vi "Autonomous Independent.vi"() -> ()   [LabVIEW 2014]
doc: "This VI is called when autonomous begins, and will automatically be terminated when autonomous ends. You can carry out timed or sensor driven robot movement independently without needing to return to the caller."
uses:
  <vilib>/Rock Robotics/WPI/CAN/TalonSRX/WPI_CANTalonSRX_APIControlMode.ctl
  <vilib>/Rock Robotics/WPI/Joystick/WPI_JoystickGetSetRefNum.vi
  Robot Global Data.vi
  <vilib>/Rock Robotics/WPI/RobotDrive/WPI_RobotDriveArcadeDrive_Standard(NoSaturation).vi
panel:
  out "Applied Throttle 2":dbl[](graph)
  out "Encoder Graph 2":dbl[](graph)
  in  "Numeric 2":dbl=1000.0 format="%#_13g"
  in  "Numeric":dbl=1000.0 format="%#_13g"
  out "Encoder Graph":dbl[](graph)
  out "Applied Throttle":dbl[](graph)
  out "Current Movement, for debugging":T1 {"Y Joystick Value" scale=1.0..-1.0; "X Joystick Value" scale=-1.0..1.0}
  in  "Array of robot movements":T2(array[cluster]) {"Y Joystick Value" scale=1.0..-1.0; "X Joystick Value" scale=-1.0..1.0}
  # "Be sure to right-click and choose Data Operations>>Make Current Value default if you want to save the array values with the VI"
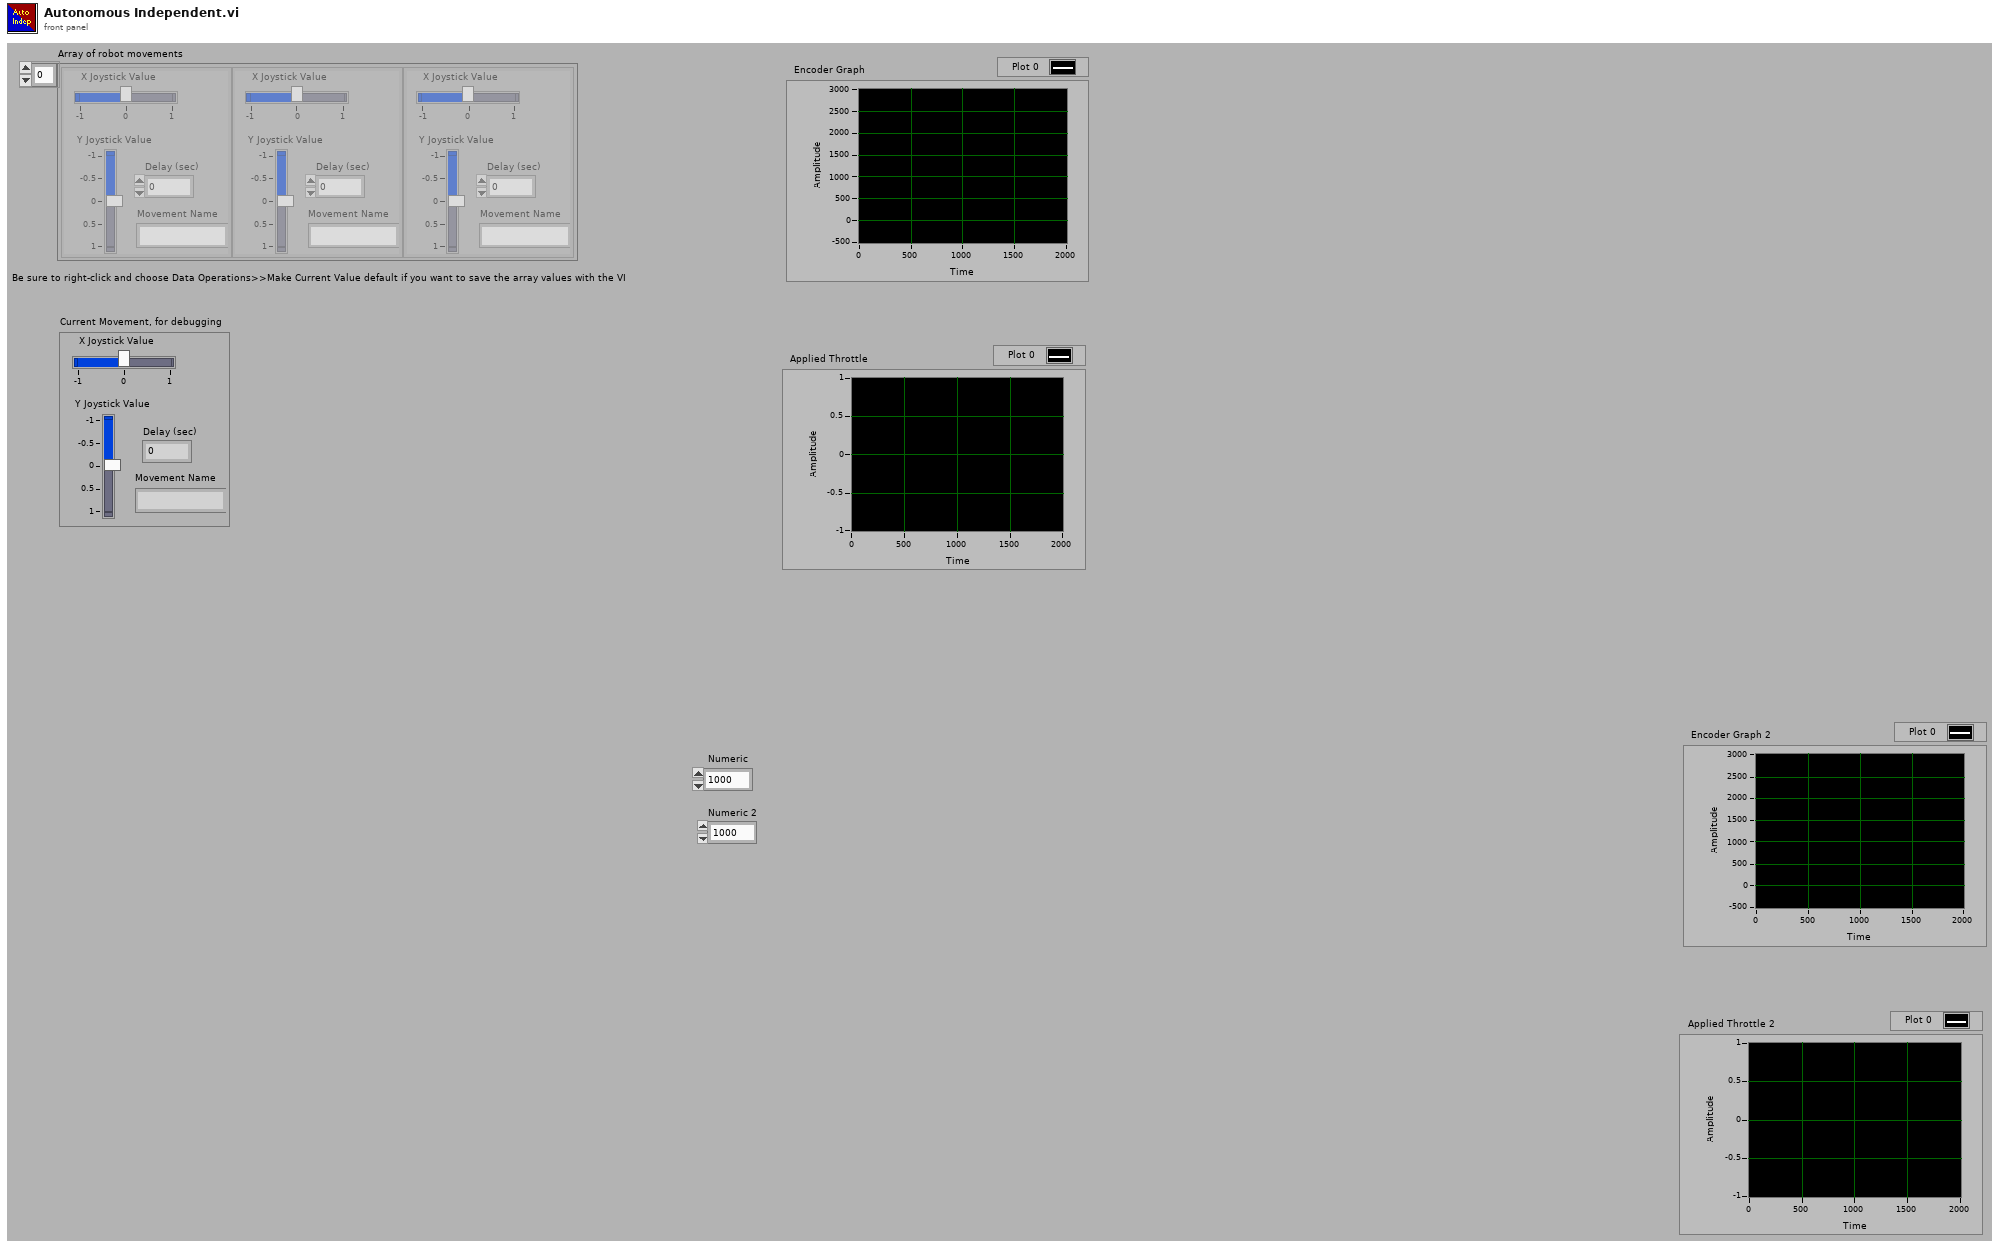
[diagram p1: front panel]
types:
  T1 = cluster{"X Joystick Value":dbl, "Y Joystick Value":dbl, "Delay (sec)":dbl, "Movement Name":string}
  T2 = cluster{"X Joystick Value":dbl, "Y Joystick Value":dbl, "Delay (sec)":dbl, "Movement Name":string}[]
  T3 = typedef "WPI_CANTalonSRX_APIControlMode.ctl" = enum8{"Percent VBus", "Speed", "Position", "Slave", "Unchanged / Invalid"}
  T4 = cluster{"proportional gain (Kc)":dbl, "integral time (Ti, min)":dbl, "derivative time (Td, min)":dbl}
  T5 = typedef "WPI_MotorControlDeviceRef.ctl" = cluster{"DeviceStatus":errorcluster, "Type":T6, "PWM":cluster{"Controller":T7, "PWM Channel":T8, "DeadBand":T9}, "CAN":cluster{"Device Number":u8, "Control Mode":T10, "Semaphore":T11, "Max Vout":dbl, "TalonSRX Control Mode":T3}, "Invert":bool, "TransformRef":T12, "InvTransformRef":T12}
  T6 = typedef "WPI_MotorControlType.ctl" = enum16{"PWM", "CAN", "CANTalonSRX"}
  T7 = typedef "FPGA_TypedefDigitalModule.ctl" = enum16{"Controller 1"}
  T8 = typedef "FPGA_DIOPWMChannel.ctl" = enum8{"PWM 0", "PWM 1", "PWM 2", "PWM 3", "PWM 4", "PWM 5", "PWM 6", "PWM 7", "PWM 8", "PWM 9", "PWM MXP 0", "PWM MXP 1", "PWM MXP 2", "PWM MXP 3", "PWM MXP 4", "PWM MXP 5", "PWM MXP 6", "PWM MXP 7", "PWM MXP 8", "PWM MXP 9", "Invalid"}
  T9 = typedef "WPI_PWMDeadband.ctl" = cluster{"Name":string, "maxPositivePwm":i32, "minPositivePwm":i32, "centerPwm":i32, "maxNegativePwm":i32, "minNegativePwm":i32, "angularRange":u16}
  T10 = typedef "WPI_CANJaguar_ControlMode.ctl" = enum8{"Percent VBus", "Current", "Speed", "Position", "Voltage"}
  T11 = typedef "Semaphore RefNum" = refnum<k1>
  T12 = typedef "WPI_PWMTransform_ConPane.ctl" = refnum<vi>
  T13 = typedef "WPI_CANTalonSRX_GlobalStatus.ctl" = cluster{"Applied Throttle":dbl, "Module Enabled":bool, "CAN Error":errorcluster, "Closed Loop Error":dbl, "Forward Limit Switch Closed":bool, "Reverse Limit Switch Closed":bool, "Sensor Position":dbl, "Sensor Velocity":dbl, "Current":dbl, "Sticky Fault - Over Temp":bool, "Sticky Fault - Under Voltage":bool, "Sticky Fault - Forward Limit":bool, "Sticky Fault - Reverse Limit":bool, "Sticky Fault - Forward Soft Limit":bool, "Sticky Fault - Reverse Soft Limit":bool, "Brake is Enabled":bool, "Encoder Position":dbl, "Encoder Velocity":dbl, "Encoder Index Count":dbl, "Encoder A Pin State":bool, "Encoder B Pin State":bool, "Encoder Index Pin State":bool, "Analog In":dbl, "Analog In Velocity":dbl, "Temperature (C)":dbl, "Battery Voltage":dbl}
  T14 = typedef "WPI_RobotDriveDevRef.ctl" = cluster{"DevStatus":errorcluster, "Motors[]":T5[], "Square Inputs":bool, "Max Output":dbl}
  T15 = typedef "WPI_EncoderDevRef.ctl" = cluster{"DevStatus":errorcluster, "EncoderIndex":T16, "CounterIndex":T17, "DistancePerCount":dbl, "Decoding Type":T18}
  T16 = typedef "FPGA_EncoderIdx.ctl" = enum8{"Enc 0", "Enc 1", "Enc 2", "Enc 3", "Enc 4", "Enc 5", "Enc 6", "Enc 7", "Invalid"}
  T17 = typedef "FPGA_CounterCtrSystemIndex.ctl" = enum8{"Ctr 0", "Ctr 1", "Ctr 2", "Ctr 3", "Ctr 4", "Ctr 5", "Ctr 6", "Ctr 7", "Invalid"}
  T18 = typedef "WPI_EncoderType.ctl" = enum16{"1x", "2x", "4x"}
  T19 = typedef "WPI_JoystickDevRef.ctl" = cluster{"Device":T20}
  T20 = typedef "WPI_JoystickDeviceEnum.ctl" = enum16{"USB 0", "USB 1", "USB 2", "USB 3", "USB 4", "USB 5"}
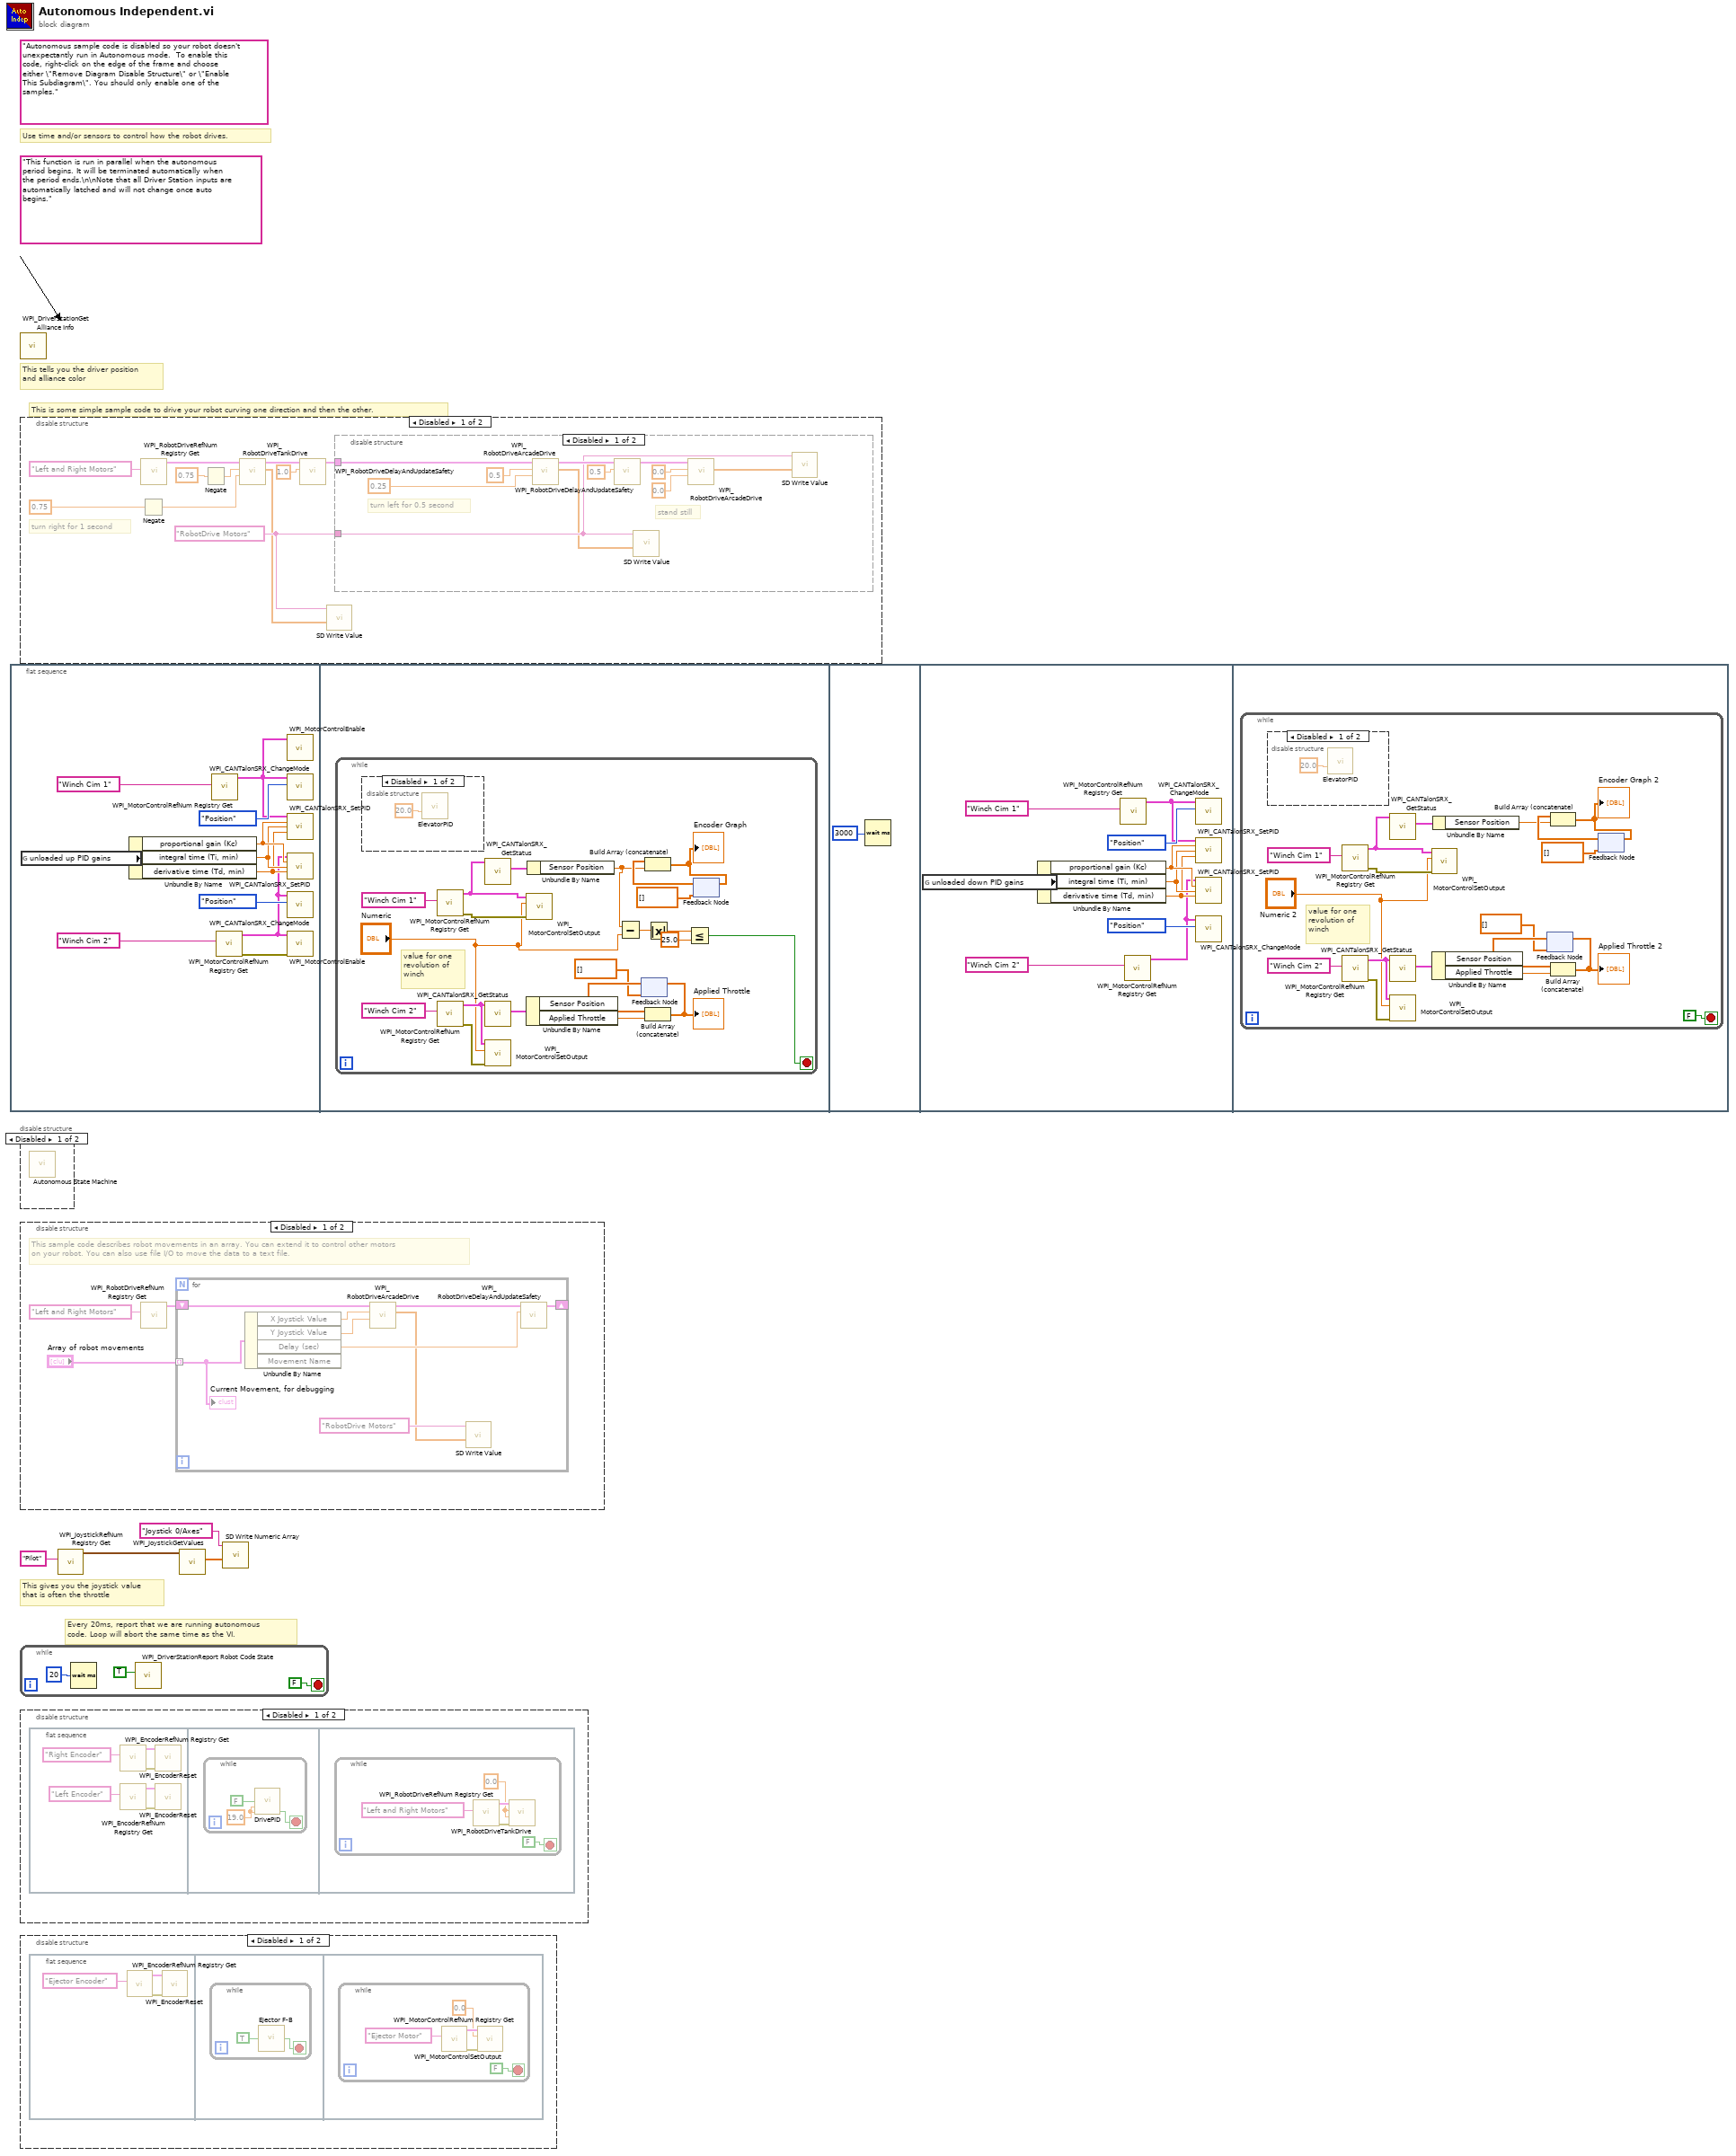
[diagram p0: block diagram]
diagram:
  (unwired) "Autonomous sample code is disabled so your robot doesn't unexpectantly run in Autonomous mode.  To enable this code, right-click on the edge of the frame and choose either \"Remove Diagram Disable Structure\" or \"Enable This Subdiagram\". You should only enable one of the samples."
  (unwired) "This function is run in parallel when the autonomous period begins. It will be terminated automatically when the period ends.\n\nNote that all Driver Station inputs are automatically latched and will not change once auto begins."
  # "This is some simple sample code to drive your robot curving one direction and then the other."
  # "Every 20ms, report that we are running autonomous\ncode. Loop will abort the same time as the VI."
  # "This gives you the joystick value\nthat is often the throttle"
  # "Use time and/or sensors to control how the robot drives."
  # "This tells you the driver position\nand alliance color"
  n1 = flat-sequence {
    frame #0 {
      n2 = global read "Robot Global Data.vi" "unloaded up PID gains"() -> (w10:T4)
      n3 = Unbundle By Name(w10) -> ("proportional gain (Kc)"=w9:dbl, "integral time (Ti, min)"=w8:dbl, "derivative time (Td, min)"=w7:dbl)
      n4 = call <vilib>:"WPI_MotorControlRefNum Registry Get.vi"("refnum name"="Winch Cim 1") -> ("MotorControlDevRef"=w5:T5)  [unwired: 9 in, 1 out]
      n5 = call <vilib>:"WPI_MotorControlRefNum Registry Get.vi"("refnum name"="Winch Cim 2") -> ("error out"=w14:errorcluster, "MotorControlDevRef"=w6:T5)  [unwired: 9 in]
      n6 = call <vilib>:"WPI_MotorControlEnable.vi"("CAN Jaguar Ref"=w5) -> ()  [unwired: 9 in, 2 out]
      n7 = call <vilib>:"WPI_CANTalonSRX_ChangeMode.vi"("Control Mode"=WPI_CANTalonSRX_APIControlMode."Position", "CAN Talon SRX Ref"=w5) -> ()  [unwired: 8 in, 2 out]
      n8 = call <vilib>:"WPI_CANTalonSRX_SetPID.vi"("CAN Talon SRX Ref"=w5, "P"=w9, "I"=w8, "D"=w7) -> ()  [unwired: 10 in, 2 out]
      n9 = call <vilib>:"WPI_CANTalonSRX_SetPID.vi"("CAN Talon SRX Ref"=w6, "P"=w9, "I"=w8, "D"=w7) -> ()  [unwired: 10 in, 2 out]
      n10 = call <vilib>:"WPI_CANTalonSRX_ChangeMode.vi"("Control Mode"=WPI_CANTalonSRX_APIControlMode."Position", "CAN Talon SRX Ref"=w6) -> ()  [unwired: 8 in, 2 out]
      n11 = call <vilib>:"WPI_MotorControlEnable.vi"("error in (no error)"=w14, "CAN Jaguar Ref"=w6) -> ()  [unwired: 8 in, 2 out]
    }
    frame #1 {
      n12 = while {
        stop <- w16 stop-if-true
        # "value for one \nrevolution of \nwinch"
        n13 = disable-structure shown="Disabled" {
          frame Disabled {
            n14 = call "ElevatorPID.vi"("Elevator Setpoint"=20.0 ("SetpointLeft")) -> ()  [unwired: 14 in, 1 out]
          }
          frame Enabled {
          }
        }
        n15 = call <vilib>:"WPI_MotorControlRefNum Registry Get.vi"("refnum name"="Winch Cim 1") -> ("error out"=w34:errorcluster, "MotorControlDevRef"=w32:T5)  [unwired: 9 in]
        n16 = call <vilib>:"WPI_MotorControlRefNum Registry Get.vi"("refnum name"="Winch Cim 2") -> ("error out"=w33:errorcluster, "MotorControlDevRef"=w31:T5)  [unwired: 9 in]
        n17 = call <vilib>:"WPI_CANTalonSRX_GetStatus.vi"("CAN Talon SRX Ref"=w32) -> ("Talon SRX Status"=w30:T13)  [unwired: 8 in, 2 out]
        n18 = call <vilib>:"WPI_CANTalonSRX_GetStatus.vi"("CAN Talon SRX Ref"=w31) -> ("Talon SRX Status"=w22:T13)  [unwired: 8 in, 2 out]
        n19 = call <vilib>:"WPI_MotorControlSetOutput.vi"("error in (no error)"=w33, "Output"="Numeric", "MotorControlDevRef"=w31) -> ()  [unwired: 6 in, 3 out]
        n20 = call <vilib>:"WPI_MotorControlSetOutput.vi"("error in (no error)"=w34, "Output"="Numeric", "MotorControlDevRef"=w32) -> ()  [unwired: 6 in, 3 out]
        n21 = Unbundle By Name(w22) -> ("Applied Throttle"=w24:dbl)  [unwired: 1 out]
        n22 = Unbundle By Name(w30) -> ("Sensor Position"=w21:dbl)
        n23 = Subtract(x=w21, y="Numeric") -> (x-y=w19:dbl)
        n24 = feedback #1(dbl[] []) -> (w29:dbl[])
        n25 = Build Array (concatenate)(w29, w24) -> (w23:dbl[])
        "Applied Throttle" <- w23
        n26 = feedback-in #1(w23) -> ()
        n27 = Absolute Value(x=w19) -> (abs(x)=w18:dbl)
        n28 = Less Or Equal?(x=w18, y=25.0) -> (x <= y?=w16:bool)
        n29 = feedback #2(dbl[] []) -> (w26:dbl[])
        n30 = Build Array (concatenate)(w26, w21) -> (w27:dbl[])
        "Encoder Graph" <- w27
        n31 = feedback-in #2(w27) -> ()
      }
    }
    frame #2 {
      n32 = Wait (ms)(milliseconds to wait=u32 3000) -> ()  [unwired: 1 out]
    }
    frame #3 {
      n33 = global read "Robot Global Data.vi" "unloaded down PID gains"() -> (w44:T4)
      n34 = Unbundle By Name(w44) -> ("proportional gain (Kc)"=w43:dbl, "integral time (Ti, min)"=w42:dbl, "derivative time (Td, min)"=w41:dbl)
      n35 = call <vilib>:"WPI_MotorControlRefNum Registry Get.vi"("refnum name"="Winch Cim 1") -> ("MotorControlDevRef"=w39:T5)  [unwired: 9 in, 1 out]
      n36 = call <vilib>:"WPI_MotorControlRefNum Registry Get.vi"("refnum name"="Winch Cim 2") -> ("MotorControlDevRef"=w40:T5)  [unwired: 9 in, 1 out]
      n37 = call <vilib>:"WPI_CANTalonSRX_ChangeMode.vi"("Control Mode"=WPI_CANTalonSRX_APIControlMode."Position", "CAN Talon SRX Ref"=w39) -> ()  [unwired: 8 in, 2 out]
      n38 = call <vilib>:"WPI_CANTalonSRX_SetPID.vi"("CAN Talon SRX Ref"=w39, "P"=w43, "I"=w42, "D"=w41) -> ()  [unwired: 10 in, 2 out]
      n39 = call <vilib>:"WPI_CANTalonSRX_SetPID.vi"("CAN Talon SRX Ref"=w40, "P"=w43, "I"=w42, "D"=w41) -> ()  [unwired: 10 in, 2 out]
      n40 = call <vilib>:"WPI_CANTalonSRX_ChangeMode.vi"("Control Mode"=WPI_CANTalonSRX_APIControlMode."Position", "CAN Talon SRX Ref"=w40) -> ()  [unwired: 8 in, 2 out]
    }
    frame #4 {
      n41 = while {
        stop <- FALSE stop-if-true
        # "value for one \nrevolution of \nwinch"
        n42 = disable-structure shown="Disabled" {
          frame Disabled {
            n43 = call "ElevatorPID.vi"("Elevator Setpoint"=20.0 ("SetpointLeft")) -> ()  [unwired: 14 in, 1 out]
          }
          frame Enabled {
          }
        }
        n44 = call <vilib>:"WPI_MotorControlRefNum Registry Get.vi"("refnum name"="Winch Cim 1") -> ("error out"=w63:errorcluster, "MotorControlDevRef"=w61:T5)  [unwired: 9 in]
        n45 = call <vilib>:"WPI_MotorControlRefNum Registry Get.vi"("refnum name"="Winch Cim 2") -> ("error out"=w62:errorcluster, "MotorControlDevRef"=w60:T5)  [unwired: 9 in]
        n46 = call <vilib>:"WPI_CANTalonSRX_GetStatus.vi"("CAN Talon SRX Ref"=w61) -> ("Talon SRX Status"=w59:T13)  [unwired: 8 in, 2 out]
        n47 = call <vilib>:"WPI_CANTalonSRX_GetStatus.vi"("CAN Talon SRX Ref"=w60) -> ("Talon SRX Status"=w51:T13)  [unwired: 8 in, 2 out]
        n48 = call <vilib>:"WPI_MotorControlSetOutput.vi"("error in (no error)"=w62, "Output"="Numeric 2", "MotorControlDevRef"=w60) -> ()  [unwired: 6 in, 3 out]
        n49 = call <vilib>:"WPI_MotorControlSetOutput.vi"("error in (no error)"=w63, "Output"="Numeric 2", "MotorControlDevRef"=w61) -> ()  [unwired: 6 in, 3 out]
        n50 = Unbundle By Name(w51) -> ("Applied Throttle"=w53:dbl)  [unwired: 1 out]
        n51 = Unbundle By Name(w59) -> ("Sensor Position"=w50:dbl)
        n52 = feedback #3(dbl[] []) -> (w58:dbl[])
        n53 = Build Array (concatenate)(w58, w53) -> (w52:dbl[])
        "Applied Throttle 2" <- w52
        n54 = feedback-in #3(w52) -> ()
        n55 = feedback #4(dbl[] []) -> (w55:dbl[])
        n56 = Build Array (concatenate)(w55, w50) -> (w56:dbl[])
        "Encoder Graph 2" <- w56
        n57 = feedback-in #4(w56) -> ()
      }
    }
  }
  n58 = call <vilib>:"WPI_DriverStationGet Alliance Info.vi"() -> ()  [unwired: 12 out]
  n59 = disable-structure shown="Disabled" {
    frame Disabled {
      w71 = "RobotDrive Motors" ("Name")
      # "turn right for 1 second"
      n60 = Negate(x=0.75 ("X axis value")) -> (-x=w68:dbl)
      n61 = call <vilib>:"WPI_RobotDriveRefNum Registry Get.vi"("refnum name"="Left and Right Motors") -> ("RobotDriveDevRef"=w72:T14)  [unwired: 1 in, 9 out]
      n62 = Negate(x=0.75 ("X axis value")) -> (-x=w69:dbl)
      n63 = call <vilib>:"WPI_RobotDriveTankDrive.vi"("Right axis value"=w68, "Left axis value"=w69, "RobotDriveDevRef"=w72) -> ("Motor Values"=w70:dbl[], "RobotDriveDevRef"=w76:T14)  [unwired: 6 in, 1 out]
      n64 = call <vilib>:"WPI_RobotDriveDelayAndUpdateSafety.vi"("Delay (s)"=1.0, "RobotDriveDevRef"=w76) -> ("RobotDriveDevRef 2"=w75:T14)  [unwired: 8 in, 1 out]
      n65 = call-poly <vilib>:"SD Write Value.vi"("Numeric Array"=w70, "Name"=w71) -> ()  [unwired: 8 in, 2 out]
      n66 = disable-structure shown="Disabled" {
        disable-tunnel: w75 -> [w85 _]
        disable-tunnel: w71 -> [w81 _]
        frame Disabled {
          # "stand still"
          # "turn left for 0.5 second"
          n67 = call-poly <vilib>:"WPI_RobotDriveArcadeDrive.vi"("Y axis value"=0.25 ("X axis value"), "X axis value"=0.5, "RobotDriveDevRef"=w85) -> ("Motor Values"=w80:dbl[], "RobotDriveDevRef"=w84:T14)  [unwired: 1 in, 6 out]
          n68 = call <vilib>:"WPI_RobotDriveDelayAndUpdateSafety.vi"("Delay (s)"=0.5, "RobotDriveDevRef"=w84) -> ("RobotDriveDevRef 2"=w83:T14)  [unwired: 8 in, 1 out]
          n69 = call-poly <vilib>:"SD Write Value.vi"("Numeric Array"=w80, "Name"=w81) -> ()  [unwired: 8 in, 2 out]
          n70 = call-poly <vilib>:"WPI_RobotDriveArcadeDrive.vi"("Y axis value"=0.0 ("X axis value"), "X axis value"=0.0, "RobotDriveDevRef"=w83) -> ("Motor Values"=w79:dbl[])  [unwired: 1 in, 7 out]
          n71 = call-poly <vilib>:"SD Write Value.vi"("Numeric Array"=w79, "Name"=w81) -> ()  [unwired: 8 in, 2 out]
        }
        frame Enabled {
        }
      }
    }
    frame Enabled {
    }
  }
  n72 = disable-structure shown="Disabled" {
    frame Disabled {
      n73 = call "Autonomous State Machine.vi"() -> ()  [unwired: 1 in]
    }
    frame Enabled {
    }
  }
  n74 = disable-structure shown="Disabled" {
    frame Disabled {
      # "This sample code describes robot movements in an array. You can extend it to control other motors\non your robot. You can also use file I/O to move the data to a text file."
      n75 = call <vilib>:"WPI_RobotDriveRefNum Registry Get.vi"("refnum name"="Left and Right Motors") -> ("RobotDriveDevRef"=w91:T14)  [unwired: 1 in, 9 out]
      n76 = for {
        shift-right: [w98] -> _
        shift-left: w91 -> [w99]
        tunnel: "Array of robot movements" -> [w94] mode=indexing
        n77 = Unbundle By Name(w94) -> ("X Joystick Value"=w97:dbl, "Y Joystick Value"=w96:dbl, "Delay (sec)"=w95:dbl)  [unwired: 1 out]
        n78 = call-poly <vilib>:"WPI_RobotDriveArcadeDrive.vi"("Y axis value"=w96, "X axis value"=w97, "RobotDriveDevRef"=w99) -> ("Motor Values"=w93:dbl[], "RobotDriveDevRef"=w100:T14)  [unwired: 1 in, 6 out]
        n79 = call-poly <vilib>:"SD Write Value.vi"("Numeric Array"=w93, "Name"="RobotDrive Motors") -> ()  [unwired: 8 in, 2 out]
        n80 = call <vilib>:"WPI_RobotDriveDelayAndUpdateSafety.vi"("Delay (s)"=w95, "RobotDriveDevRef"=w100) -> ("RobotDriveDevRef 2"=w98:T14)  [unwired: 8 in, 1 out]
        "Current Movement, for debugging" <- w94
      }
    }
    frame Enabled {
    }
  }
  n81 = while {
    stop <- FALSE stop-if-true
    n82 = Wait (ms)(milliseconds to wait=u32 20) -> ()  [unwired: 1 out]
    n83 = call <vilib>:"WPI_DriverStationReport Robot Code State.vi"("Autonomous"=TRUE) -> ()  [unwired: 10 in, 1 out]
  }
  n84 = disable-structure shown="Disabled" {
    frame Disabled {
      n85 = flat-sequence {
        frame #0 {
          n86 = call <vilib>:"WPI_EncoderRefNum Registry Get.vi"("refnum name"="Right Encoder") -> ("error out"=w108:errorcluster, "EncoderDevRef"=w107:T15)  [unwired: 9 in]
          n87 = call <vilib>:"WPI_EncoderRefNum Registry Get.vi"("refnum name"="Left Encoder") -> ("error out"=w110:errorcluster, "EncoderDevRef"=w109:T15)  [unwired: 9 in]
          n88 = call <vilib>:"WPI_EncoderReset.vi"("error in (no error)"=w108, "EncoderDevRef"=w107) -> ()  [unwired: 8 in, 2 out]
          n89 = call <vilib>:"WPI_EncoderReset.vi"("error in (no error)"=w110, "EncoderDevRef"=w109) -> ()  [unwired: 8 in, 2 out]
        }
        frame #1 {
          n90 = while {
            stop <- w111 stop-if-true
            w112 = 19.0 ("SetpointLeft")
            n91 = call "DrivePID.vi"("Compensate"=FALSE, "SetpointRight"=w112, "SetpointLeft"=w112) -> ("Done"=w111:bool)  [unwired: 12 in]
          }
        }
        frame #2 {
          n92 = while {
            stop <- FALSE stop-if-true
            w115 = 0.0 ("Left axis value")
            n93 = call <vilib>:"WPI_RobotDriveRefNum Registry Get.vi"("refnum name"="Left and Right Motors") -> ("error out"=w117:errorcluster, "RobotDriveDevRef"=w116:T14)  [unwired: 9 in]
            n94 = call <vilib>:"WPI_RobotDriveTankDrive.vi"("error in (no error)"=w117, "Right axis value"=w115, "Left axis value"=w115, "RobotDriveDevRef"=w116) -> ()  [unwired: 5 in, 3 out]
          }
        }
      }
    }
    frame Enabled {
    }
  }
  n95 = disable-structure shown="Disabled" {
    frame Disabled {
      n96 = flat-sequence {
        frame #0 {
          n97 = call <vilib>:"WPI_EncoderRefNum Registry Get.vi"("refnum name"="Ejector Encoder") -> ("error out"=w121:errorcluster, "EncoderDevRef"=w120:T15)  [unwired: 9 in]
          n98 = call <vilib>:"WPI_EncoderReset.vi"("error in (no error)"=w121, "EncoderDevRef"=w120) -> ()  [unwired: 8 in, 2 out]
        }
        frame #1 {
          n99 = while {
            stop <- w122 stop-if-true
            n100 = call "Ejector F-B.vi"("go to forward limit?"=TRUE ("Compensate")) -> ("Limit Reached"=w122:bool)
          }
        }
        frame #2 {
          n101 = while {
            stop <- FALSE stop-if-true
            n102 = call <vilib>:"WPI_MotorControlRefNum Registry Get.vi"("refnum name"="Ejector Motor") -> ("error out"=w127:errorcluster, "MotorControlDevRef"=w126:T5)  [unwired: 9 in]
            n103 = call <vilib>:"WPI_MotorControlSetOutput.vi"("error in (no error)"=w127, "Output"=0.0, "MotorControlDevRef"=w126) -> ()  [unwired: 6 in, 3 out]
          }
        }
      }
    }
    frame Enabled {
    }
  }
  n104 = call <vilib>:"WPI_JoystickRefNum Registry Get.vi"("refnum name"="Pilot") -> ("JoystickDevRef"=w3:T19)  [unwired: 1 in, 9 out]
  n105 = call <vilib>:"WPI_JoystickGetValues.vi"("JoystickDevRef"=w3) -> ("Axes"=w1:dbl[])  [unwired: 6 in, 4 out]
  n106 = call <vilib>:"SD Write Numeric Array.vi"("Numeric Array"=w1, "Name"="Joystick 0/Axes") -> ()  [unwired: 8 in, 2 out]
